vi "niFpgaMeanVarStdDefaultTemplate.vi"(0 "input data":fxp<+/-,16,16>, 1 "reset":bool) -> (4 "mean":fxp<+/-,16,16>, 10 "output valid":bool)   [LabVIEW 2017]
uses:
  <vilib>/Platform/TimedLoop/XDataNode/timing_clust.ctl
  <vilib>/Platform/TimedLoop/XDataNode/nitl_modes.ctl
  <vilib>/Platform/TimedLoop/XDataNode/wakeup.ctl
  <vilib>/rvi/FXPMathLib/basic elements/FxpIntAccumulator/subVIs/nifxpmath_IntAccumulator_SimConfig.ctl
  <vilib>/rvi/FXPMathLib/basic elements/FxpIntAccumulator/simVIs/DllFxpIntAccumulator_sub.vi
  <vilib>/Platform/TimedLoop/XDataNode/XDataNode.xnode
  <vilib>/rvi/FXPMathLib/basic elements/FxpIntAccumulator/XNode/nifxpmath_IntAccumulator.xnode
  <vilib>/rvi/FXPMathLib/FxpMul/XNode/nifxpmath_Multiplier.xnode
  <vilib>/Platform/TimedLoop/XDataNode/XDNodeRunTimeDep.lvlib
  <vilib>/rvi/FXPMathLib/sim/FxpSim.dll
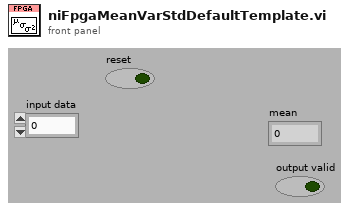
[diagram p1: front panel]
types:
  T1 = typedef "XDNodeRunTimeDep.lvlib/timing_clust.ctl" = cluster{"Expected End [f-1]":u64, "Actual End [f-1]":u64, "Finished Late? [f-1]":bool, "Expected End [i-1]":u64, "Actual End [i-1]":u64, "Finished Late? [i-1]":bool, "Expected Start [i]":u64, "Actual Start [i]":u64, "Expected Start [f]":u64, "Actual Start [f]":u64, "Source Name":string, "Structure Name":string, "Period":i64, "Deadline":i64, "Offset":i64, "Start":i64, "Priority":i32, "Timeout":i32, "Mode":T2, "Wakeup Reason":T3, "Error":errorcluster, "Source Type":string, "Secondary Source Type":string, "Global End Time":u64, "Global Start Time":u64, "Frame Duration":u64, "Iteration Duration":u64, "Assigned CPU":i32, "I/O Scan Engine Mode":u32}
  T2 = typedef "XDNodeRunTimeDep.lvlib/nitl_modes.ctl" = enum32{"No Change", "Process missed periods, maintain original phase", "Discard missed periods, maintain original phase", "Process missed periods, ignore original phase", "Discard missed periods, ignore original phase"}
  T3 = typedef "XDNodeRunTimeDep.lvlib/wakeup.ctl" = enum32{"Normal", "Aborted", "Asynchronous wakeup", "Timing source error", "Timed loop error", "Timeout"}
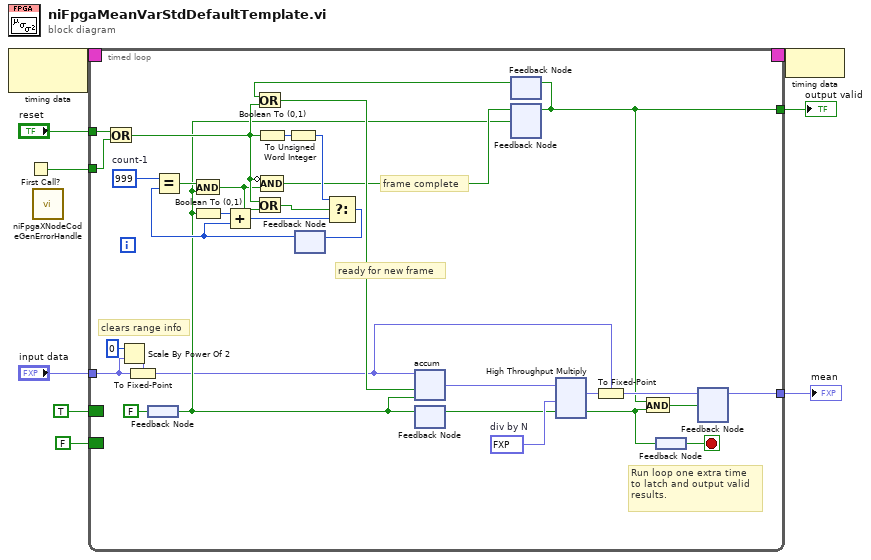
[diagram p0: block diagram]
diagram:
  n1 = node-c288() -> (w9:T1)  [unwired: 1 in]
  n2 = First Call?() -> (First Call?: T/F=w1:bool)
  n3 = call <vilib>:"niFpgaXNodeCodeGenErrorHandle.vi"() -> ()  [unwired: 1 in]
  n4 = timed-loop {
    tunnel: [w17] -> w5
    tunnel: "input data" -> [w13]
    tunnel: "reset" -> [w37]
    tunnel: w1 -> [w36]
    tunnel: [w16] -> w4
    timing: w9 -> [_]
    timing-out: [_] -> w8
    border: TRUE -> [_]
    border: FALSE ("output valid") -> [_]
    stop <- w14 stop-if-true
    w27 = fxp<+,17,-9> 0.0010000020265579224  # div by N
    w41 = u16 999  # count-1
    # "Run loop one extra time\nto latch and output valid\nresults."
    # "clears range info"
    # "frame complete"
    # "ready for new frame"
    n5 = Or(x=w37, y=w36) -> (x .or. y?=w31:bool)
    n6 = Scale By Power Of 2(n=0, x=w13) -> (x*2^n=w21:fxp<+/-,16,16>)
    n7 = To Fixed-Point(fixed-point type=w21, number=w13) -> (fixed-point=w12:fxp<+/-,16,16>)
    n8 = feedback #1() -> (w19:bool)
    n9 = feedback-in #1(FALSE) -> ()
    n10 = Boolean To (0,1)(Boolean=w19) -> (0, 1=w35:i16)
    n11 = Boolean To (0,1)(Boolean=w31) -> (0, 1=w40:i16)
    n12 = To Unsigned Word Integer(number=w40) -> (unsigned 16bit integer=w39:u16)
    n13 = feedback #2() -> (w28:u16)  [unwired: 1 in]
    n14 = Equal?(x=w41, y=w28) -> (x = y?=w33:bool)
    n15 = And(x=w33, y=w19) -> (x .and. y?=w30:bool)
    n16 = Add(x=w35, y=w28) -> (x+y=w34:u16)
    n17 = Or(x=w31, y=w30) -> (x .or. y?=w32:bool)
    n18 = Compound Arithmetic op=AND(invert w31, w30) -> (w24:bool)
    n19 = Select(t=w39, s=w32, f=w34) -> (s? t:f=w38:u16)
    n20 = feedback-in #2(w38) -> ()
    n21 = feedback-in #3(w19) -> ()
    n22 = feedback #3() -> (w23:bool)  [unwired: 1 in]
    n23 = feedback #4() -> (w29:bool)  [unwired: 1 in]
    n24 = Or(x=w29, y=w31) -> (x .or. y?=w25:bool)
    n25 = xnode "accum"("x"=w12, "load (F)"=w25, "enable (T)"=w19) -> ("s"=w26:fxp<+/-,26,26>)  [unwired: 2 in, 1 out]
    n26 = feedback-in #5(w24, w19) -> ()
    n27 = feedback #5() -> (w16:bool)  [unwired: 1 in]
    n28 = feedback-in #4(w16) -> ()
    n29 = xnode ("High Throughput Multiply")("x"=w26, "y"=w27, "input valid"=w23) -> ("x*y"=w11:fxp<+/-,43,17>, "output valid"=w10:bool)  [unwired: 1 in, 1 out]
    n30 = To Fixed-Point(fixed-point type=w12, number=w11) -> (fixed-point=w18:fxp<+/-,16,16>)
    n31 = And(x=w16, y=w10) -> (x .and. y?=w15:bool)
    n32 = feedback-in #6(w10) -> ()
    n33 = feedback #6() -> (w14:bool)
    n34 = feedback #7() -> (w17:fxp<+/-,16,16>)  [unwired: 1 in]
    n35 = feedback-in #7(w18, w15) -> ()
  }
  "mean" <- w5
  "output valid" <- w4
  n36 = node-c288(w8) -> ()
